vi "历史温度曲线.vi"   [LabVIEW 2016, in "斯坦道氨氮.lvlib"]
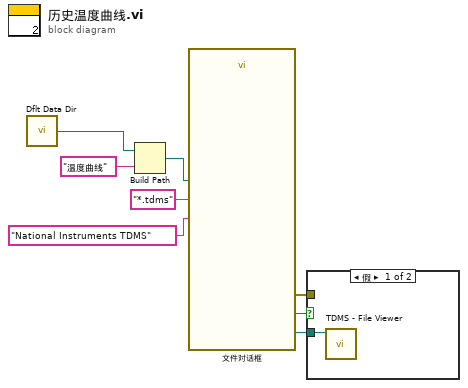
[diagram p0: block diagram]
diagram:
  n1 = call <vilib>:"Dflt Data Dir.vi"() -> ("App:Default Data Directory"=w4:path)
  n2 = Build Path(base path=w4, name or relative path="温度曲线" ("名称或相对路径")) -> (appended path=w5:path)
  n3 = call "文件对话框"("start path"=w5, "pattern (all files)"="*.tdms", "pattern label"="National Instruments TDMS") -> ("selected path"=w6:path, "cancelled"=w2:bool, "error out"=w1:errorcluster)  [unwired: 9 in, 1 out]
  n4 = case shown="假" w2 {
    tunnel: w6 -> [w9 _]
    tunnel: w1 -> [_ _]
    frame False {
      n5 = call <vilib>:"TDMS - File Viewer.vi"("file path"=w9) -> ()  [unwired: 5 in, 2 out]
    }
    frame True {
    }
  }
